vi "Clear Arbitrary Waveform [ARB].vi"(8 "error in (no error)":errorcluster, 10 "waveform handle (0)":i32, 11 "CS++Fgen in":refnum<class "CS++Fgen.lvclass">) -> (0 "error out":errorcluster, 3 "CS++Fgen out":refnum<class "CS++Fgen.lvclass">)   [LabVIEW 2013, in "CS++Fgen.lvlib" / "CS++Fgen.lvclass"]
doc: "This VI removes a previously created arbitrary waveform from the function generator's memory and invalidates the waveform's handle.\n\nNotes:\n\n(1) This VI is part of the IviFgenArbWfm [ARB] extension group."
uses:
  CS++Fgen.lvclass
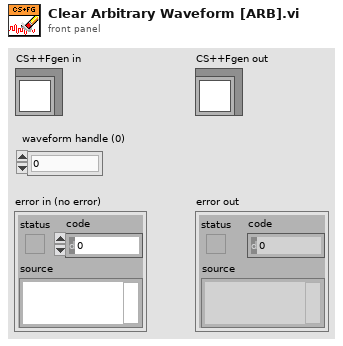
[diagram p1: front panel]
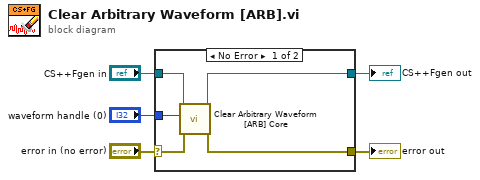
[diagram p0: block diagram]
diagram:
  n1 = case shown="No Error" "error in (no error)" {
    selector: "error in (no error)" -> [w8 w12]
    tunnel: [w7 w12] -> w4
    tunnel: [w9 w11] -> w2
    tunnel: "CS++Fgen in" -> [w10 w11]
    tunnel: "waveform handle (0)" -> [w6 _]
    frame No Error {
      n2 = call-dynamic "Clear Arbitrary Waveform [ARB] Core.vi"("error in (no error)"=w8, "waveform handle (0)"=w6, "CS++Fgen in"=w10) -> ("error out"=w7:errorcluster, "CS++Fgen out"=w9:refnum<class "CS++Fgen.lvclass">)  [unwired: 7 in]
    }
    frame Error {
    }
  }
  "error out" <- w4
  "CS++Fgen out" <- w2
